vi "HighSpeedInit.vi"(8 "error in":errorcluster, 10 "Fast":bool=TRUE, 11 "VISA Refnum in":refnum<visa-resource-name>) -> (0 "error out":errorcluster, 3 "VISA Refnum out":refnum<visa-resource-name>)   [LabVIEW 2016]
uses:
  <vilib>/Instr/_visa.llb/VISA Configure Serial Port (Instr).vi
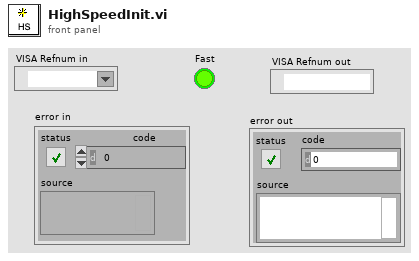
[diagram p1: front panel]
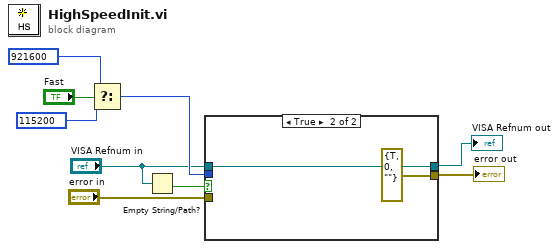
[diagram p0: block diagram]
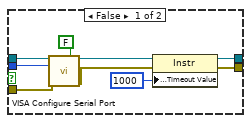
[diagram p2: hidden frame]
diagram:
  n1 = Select(t=u32 921600 ("baud rate (115200)"), s="Fast", f=u32 115200 ("baud rate (115200)")) -> (s? t:f=w3:u32)
  n2 = Empty String/Path?(string/path="VISA Refnum in") -> (empty?=w1:bool)
  n3 = case shown="True" w1 {
    tunnel: [w18 w20] -> w9
    tunnel: "error in" -> [w14 _]
    tunnel: [w12 errorcluster {"status"=TRUE, "code"=0, "source"=""} ("error out")] -> w7
    tunnel: w3 -> [w11 _]
    tunnel: "VISA Refnum in" -> [w10 w20]
    frame False {
      n4 = call-poly "VISA Configure Serial Port"("VISA resource name"=w10, "Enable Termination\nChar (T)"=FALSE ("Enable Termination\nChar (T)"), "baud rate (9600)"=w11, "error in (no error)"=w14) -> ("VISA resource name out"=w17:refnum<visa-resource-name>, "error out"=w13:errorcluster)  [unwired: 10 in]
      n5 = property class="Instr"(reference=w17, error in=w13, "General Settings:Timeout Value"=u32 1000) -> (reference out=w18:refnum<visa-resource-name>, error out=w12:errorcluster)
    }
    frame True {
    }
  }
  "VISA Refnum out" <- w9
  "error out" <- w7
